vi "EventSignalToRingCtrl.vi"(11 "ref in":refnum<vi>) -> (2 "out":i32, 3 "ref out":refnum<vi>)   [LabVIEW 2018, in "Library-Ctrl.lvlib"]
uses:
  Library-Ctrl.lvlib
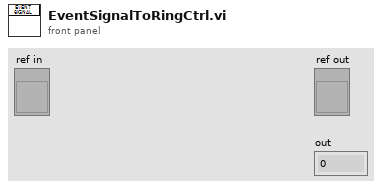
[diagram p1: front panel]
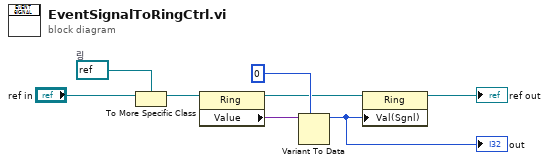
[diagram p0: block diagram]
diagram:
  w7 = refnum<vi> refnum  # 링
  n1 = To More Specific Class(target class=w7, reference="ref in") -> (specific class reference=w6:refnum<vi>)  [unwired: 1 in, 1 out]
  n2 = property class="Ring"(reference=w6) -> (reference out=w3:refnum<vi>, "Value"=w5:variant)  [unwired: 1 in, 1 out]
  n3 = Variant To Data(type=0, Variant=w5) -> (data=w1:i32)  [unwired: 1 in, 1 out]
  "out" <- w1
  n4 = property class="Ring"(reference=w3, "Val(Sgnl)"=w1) -> (reference out=→"ref out":refnum<vi>)  [unwired: 1 in, 1 out]
